vi "Save Output (SubVI).vi"(0 "Contour Array":cluster{"Array":i32[], "Array":i32[]}[](array[cluster]), 2 "SPINE Array":cluster{"Array":dbl[], "Array":dbl[]}[](array[cluster]), 3 "date/time string":string, 4 "Larvae ID":u32[](array[numeric]), 5 "Data":T1, 7 "Contour REF In":refnum<file>, 8 "Pixel Resolution (um/Pixel)":dbl=0.04069 format="%#_13g", 9 "SPINE REF In":refnum<file>) -> (11 "Contour REF Out":refnum<file>, 13 "SPINE REF Out":refnum<file>)   [LabVIEW 2015]
uses:
  Controls (HOST)/Data to Disk Bundle.ctl
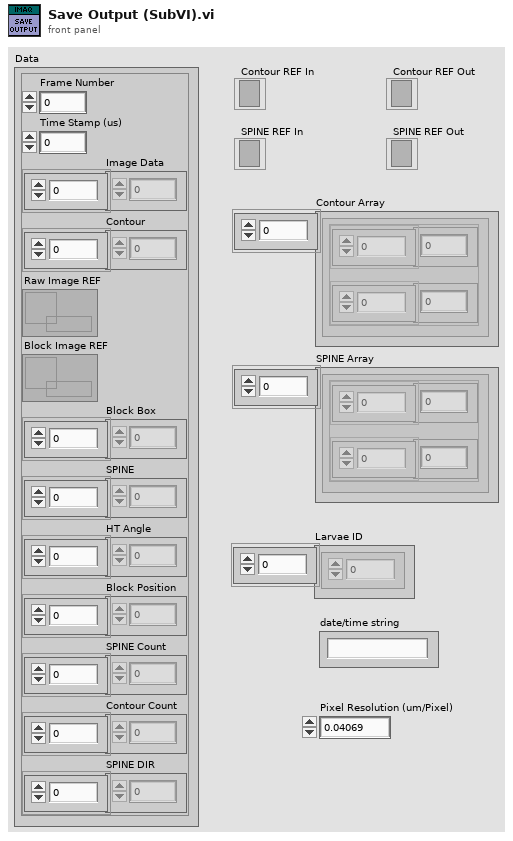
[diagram p1: front panel]
types:
  T1 = typedef "Data to Disk Bundle.ctl" = cluster{"Frame Number":u64, "Time Stamp (us)":u64, "Image Data":u64[], "Contour":u32[], "Raw Image REF":refnum<data-value>, "Block Image REF":refnum<data-value>, "Block Box":u64[], "SPINE":u32[], "HT Angle":u64[], "Block Position":u64[], "SPINE Count":u32[], "Contour Count":u32[], "SPINE DIR":u8[]}
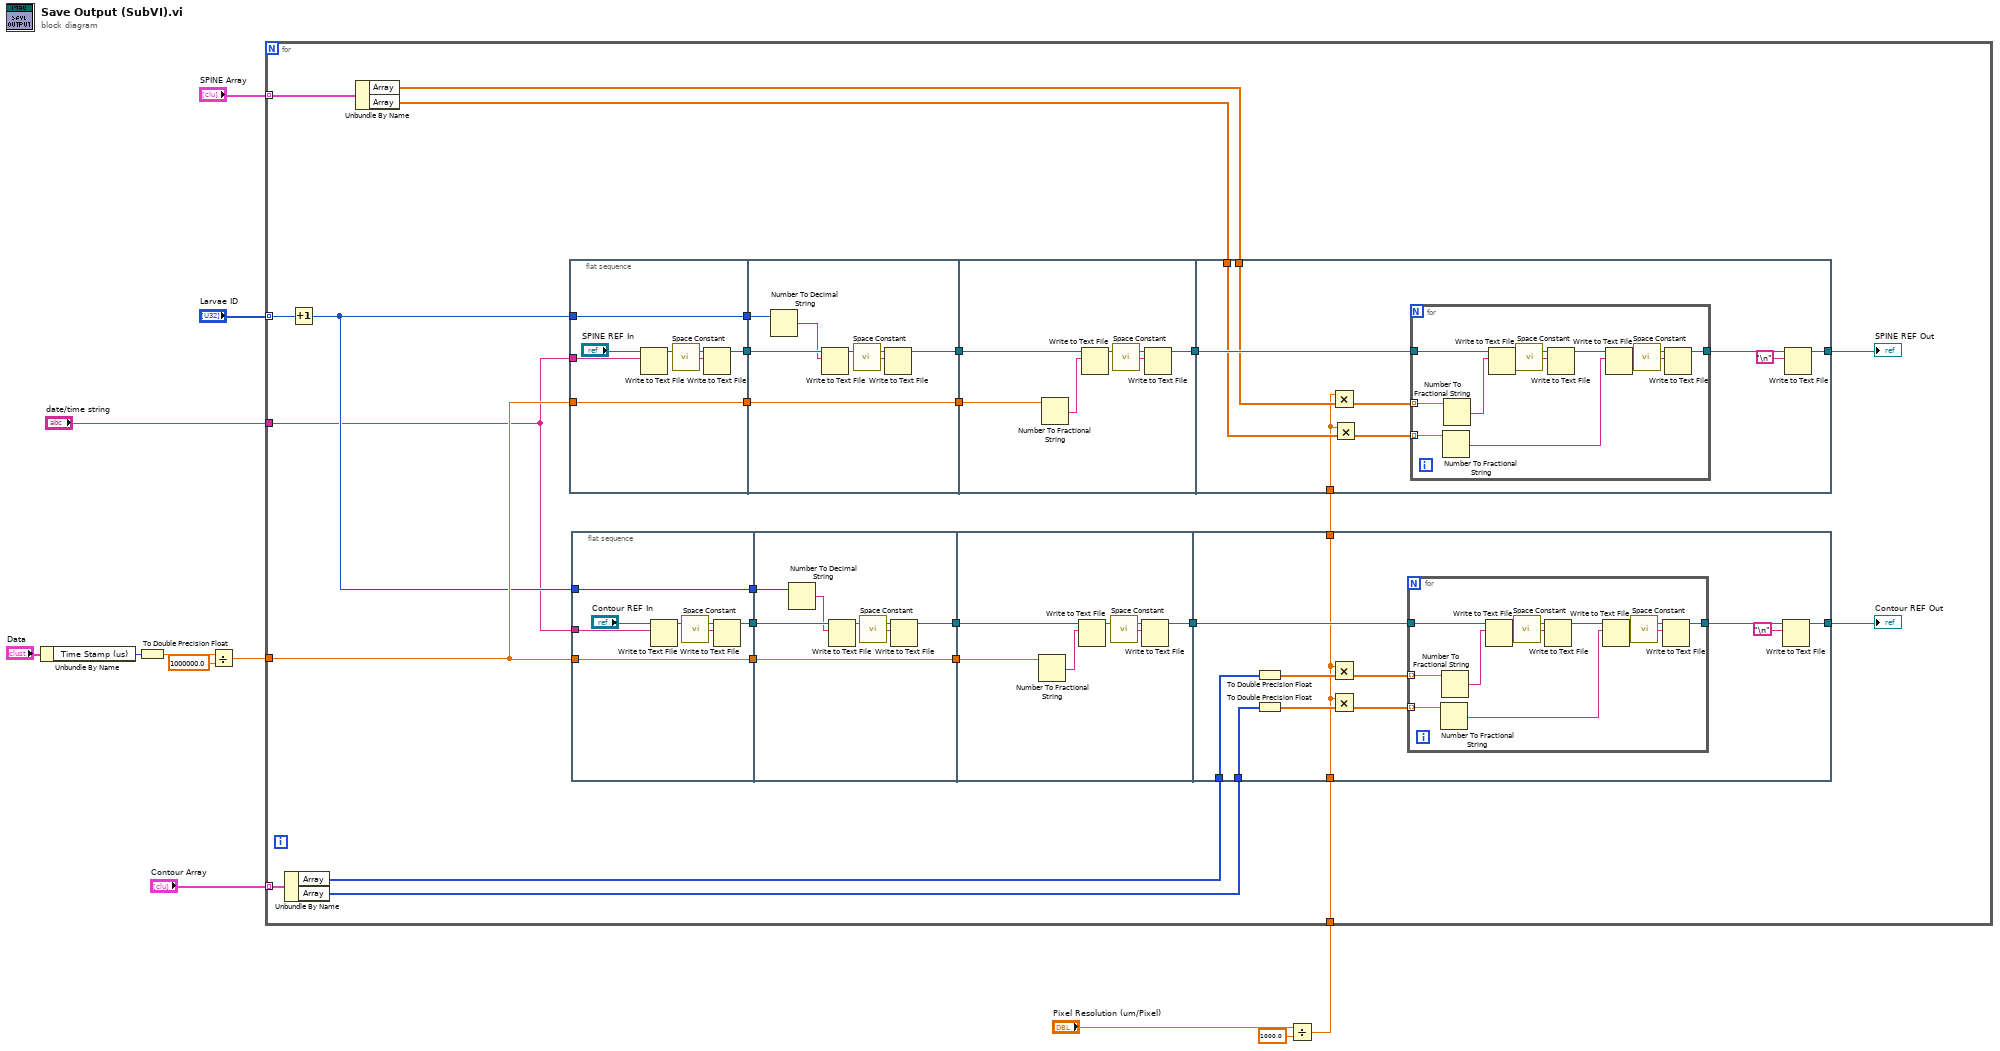
[diagram p0: block diagram]
diagram:
  n1 = Unbundle By Name("Data") -> ("Time Stamp (us)"=w8:u64)
  n2 = To Double Precision Float(number=w8) -> (double precision float=w7:dbl)
  n3 = Divide(x=w7, y=1000000.0 ("x")) -> (x/y=w6:dbl)
  n4 = Divide(x="Pixel Resolution (um/Pixel)", y=1000.0 ("x")) -> (x/y=w2:dbl)
  n5 = for {
    tunnel: "SPINE Array" -> [w38] mode=indexing
    tunnel: "Larvae ID" -> [w31] mode=indexing
    tunnel: w6 -> [w35]
    tunnel: "Contour Array" -> [w34] mode=indexing
    tunnel: "date/time string" -> [w29]
    tunnel: w2 -> [w28]
    n6 = Unbundle By Name(w34) -> ("Array"=w33:i32[], "Array"=w32:i32[])
    n7 = Increment(x=w31) -> (x+1=w30:u32)
    n8 = Unbundle By Name(w38) -> ("Array"=w36:dbl[], "Array"=w37:dbl[])
    n9 = flat-sequence {
      tunnel: [w85] -> w27
      tunnel: w30 -> [w83]
      tunnel: [w83] -> w26
      tunnel: w29 -> [w82]
      tunnel: w35 -> [w81]
      tunnel: [w81] -> w25
      tunnel: w27 -> [w92]
      tunnel: [w91] -> w24
      tunnel: w26 -> [w89]
      tunnel: [w88] -> w23
      tunnel: w25 -> [w88]
      tunnel: w24 -> [w98]
      tunnel: [w96] -> w22
      tunnel: w23 -> [w95]
      tunnel: w22 -> [w109]
      tunnel: [w106] -> w15
      tunnel: w36 -> [w105]
      tunnel: w37 -> [w104]
      tunnel: w13 -> [w101]
      frame #0 {
        n10 = Write to Text File(file (use dialog)="SPINE REF In", text=w82) -> (refnum out=w87:refnum<file>)  [unwired: 2 in, 2 out]
        n11 = call <vilib>:"Space Constant.vi"() -> ("String"=w86:string)
        n12 = Write to Text File(file (use dialog)=w87, text=w86) -> (refnum out=w85:refnum<file>)  [unwired: 2 in, 2 out]
      }
      frame #1 {
        n13 = Number To Decimal String(number=w89) -> (decimal integer string=w90:string)  [unwired: 1 in]
        n14 = Write to Text File(file (use dialog)=w92, text=w90) -> (refnum out=w93:refnum<file>)  [unwired: 2 in, 2 out]
        n15 = call <vilib>:"Space Constant.vi"() -> ("String"=w94:string)
        n16 = Write to Text File(file (use dialog)=w93, text=w94) -> (refnum out=w91:refnum<file>)  [unwired: 2 in, 2 out]
      }
      frame #2 {
        n17 = Number To Fractional String(number=w95) -> (F-format string=w97:string)  [unwired: 3 in]
        n18 = Write to Text File(file (use dialog)=w98, text=w97) -> (refnum out=w100:refnum<file>)  [unwired: 2 in, 2 out]
        n19 = call <vilib>:"Space Constant.vi"() -> ("String"=w99:string)
        n20 = Write to Text File(file (use dialog)=w100, text=w99) -> (refnum out=w96:refnum<file>)  [unwired: 2 in, 2 out]
      }
      frame #3 {
        n21 = Multiply(x=w101, y=w105) -> (x*y=w103:dbl[])
        n22 = Multiply(x=w101, y=w104) -> (x*y=w102:dbl[])
        n23 = for {
          tunnel: w109 -> [w120]
          tunnel: w103 -> [w117] mode=indexing
          tunnel: w102 -> [w110] mode=indexing
          tunnel: [w112] -> w107
          n24 = Number To Fractional String(number=w110) -> (F-format string=w111:string)  [unwired: 3 in]
          n25 = Number To Fractional String(number=w117) -> (F-format string=w116:string)  [unwired: 3 in]
          n26 = Write to Text File(file (use dialog)=w120, text=w116) -> (refnum out=w118:refnum<file>)  [unwired: 2 in, 2 out]
          n27 = call <vilib>:"Space Constant.vi"() -> ("String"=w119:string)
          n28 = Write to Text File(file (use dialog)=w118, text=w119) -> (refnum out=w113:refnum<file>)  [unwired: 2 in, 2 out]
          n29 = Write to Text File(file (use dialog)=w113, text=w111) -> (refnum out=w115:refnum<file>)  [unwired: 2 in, 2 out]
          n30 = call <vilib>:"Space Constant.vi"() -> ("String"=w114:string)
          n31 = Write to Text File(file (use dialog)=w115, text=w114) -> (refnum out=w112:refnum<file>)  [unwired: 2 in, 2 out]
        }
        n32 = Write to Text File(file (use dialog)=w107, text="\n") -> (refnum out=w106:refnum<file>)  [unwired: 2 in, 2 out]
      }
    }
    n33 = flat-sequence {
      tunnel: [w43] -> w21
      tunnel: w30 -> [w41]
      tunnel: [w41] -> w20
      tunnel: w29 -> [w40]
      tunnel: w35 -> [w39]
      tunnel: [w39] -> w19
      tunnel: w21 -> [w50]
      tunnel: [w49] -> w18
      tunnel: w20 -> [w47]
      tunnel: [w46] -> w17
      tunnel: w19 -> [w46]
      tunnel: w18 -> [w56]
      tunnel: [w54] -> w16
      tunnel: w17 -> [w53]
      tunnel: w16 -> [w69]
      tunnel: [w66] -> w14
      tunnel: w33 -> [w65]
      tunnel: w32 -> [w64]
      tunnel: w28 -> [w59]
      tunnel: [w59] -> w13
      frame #0 {
        n34 = Write to Text File(file (use dialog)="Contour REF In", text=w40) -> (refnum out=w45:refnum<file>)  [unwired: 2 in, 2 out]
        n35 = call <vilib>:"Space Constant.vi"() -> ("String"=w44:string)
        n36 = Write to Text File(file (use dialog)=w45, text=w44) -> (refnum out=w43:refnum<file>)  [unwired: 2 in, 2 out]
      }
      frame #1 {
        n37 = Number To Decimal String(number=w47) -> (decimal integer string=w48:string)  [unwired: 1 in]
        n38 = Write to Text File(file (use dialog)=w50, text=w48) -> (refnum out=w51:refnum<file>)  [unwired: 2 in, 2 out]
        n39 = call <vilib>:"Space Constant.vi"() -> ("String"=w52:string)
        n40 = Write to Text File(file (use dialog)=w51, text=w52) -> (refnum out=w49:refnum<file>)  [unwired: 2 in, 2 out]
      }
      frame #2 {
        n41 = Number To Fractional String(number=w53) -> (F-format string=w55:string)  [unwired: 3 in]
        n42 = Write to Text File(file (use dialog)=w56, text=w55) -> (refnum out=w58:refnum<file>)  [unwired: 2 in, 2 out]
        n43 = call <vilib>:"Space Constant.vi"() -> ("String"=w57:string)
        n44 = Write to Text File(file (use dialog)=w58, text=w57) -> (refnum out=w54:refnum<file>)  [unwired: 2 in, 2 out]
      }
      frame #3 {
        n45 = To Double Precision Float(number=w65) -> (double precision float=w63:dbl[])
        n46 = To Double Precision Float(number=w64) -> (double precision float=w62:dbl[])
        n47 = Multiply(x=w59, y=w63) -> (x*y=w61:dbl[])
        n48 = Multiply(x=w59, y=w62) -> (x*y=w60:dbl[])
        n49 = for {
          tunnel: w69 -> [w80]
          tunnel: w61 -> [w77] mode=indexing
          tunnel: w60 -> [w70] mode=indexing
          tunnel: [w72] -> w67
          n50 = Number To Fractional String(number=w70) -> (F-format string=w71:string)  [unwired: 3 in]
          n51 = Number To Fractional String(number=w77) -> (F-format string=w76:string)  [unwired: 3 in]
          n52 = Write to Text File(file (use dialog)=w80, text=w76) -> (refnum out=w78:refnum<file>)  [unwired: 2 in, 2 out]
          n53 = call <vilib>:"Space Constant.vi"() -> ("String"=w79:string)
          n54 = Write to Text File(file (use dialog)=w78, text=w79) -> (refnum out=w73:refnum<file>)  [unwired: 2 in, 2 out]
          n55 = Write to Text File(file (use dialog)=w73, text=w71) -> (refnum out=w75:refnum<file>)  [unwired: 2 in, 2 out]
          n56 = call <vilib>:"Space Constant.vi"() -> ("String"=w74:string)
          n57 = Write to Text File(file (use dialog)=w75, text=w74) -> (refnum out=w72:refnum<file>)  [unwired: 2 in, 2 out]
        }
        n58 = Write to Text File(file (use dialog)=w67, text="\n") -> (refnum out=w66:refnum<file>)  [unwired: 2 in, 2 out]
      }
    }
    "SPINE REF Out" <- w15
    "Contour REF Out" <- w14
  }
